vi "authorize summary.vi"(4 "error in (no error)":errorcluster, 6 "Authorization Request Sent? (f)":bool, 7 "Authorization":T2) -> (0 "error out":errorcluster, 3 "Template Keys":T1)   [LabVIEW 2011]
uses:
  license/Authorization Data.ctl
  ITK EXT/utils/keyedarr.llb/Keyed Array.ctl
  server/server lib/Spartan CONFIG Global.vi
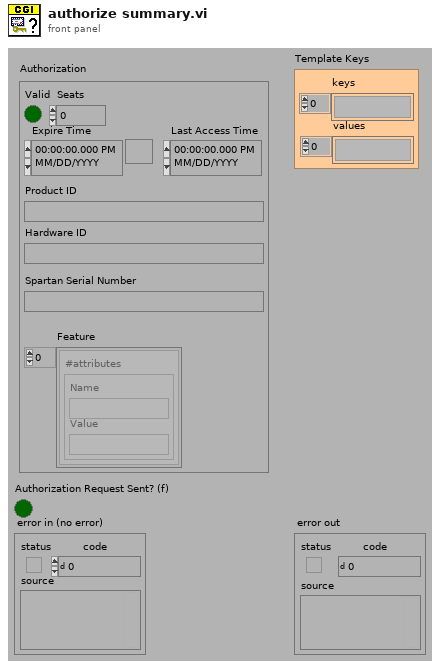
[diagram p1: front panel]
types:
  T1 = typedef "Keyed Array.ctl" = cluster{"keys":string[], "values":string[]}
  T2 = typedef "Authorization Data.ctl" = cluster{"Valid":bool, "Seats":i32, "Expire Time":timestamp, "Last Access Time":timestamp, "Product ID":string, "Hardware ID":string, "Spartan Serial Number":string, "Feature":cluster{"#attributes":cluster{"Name":string, "Value":string}}[]}
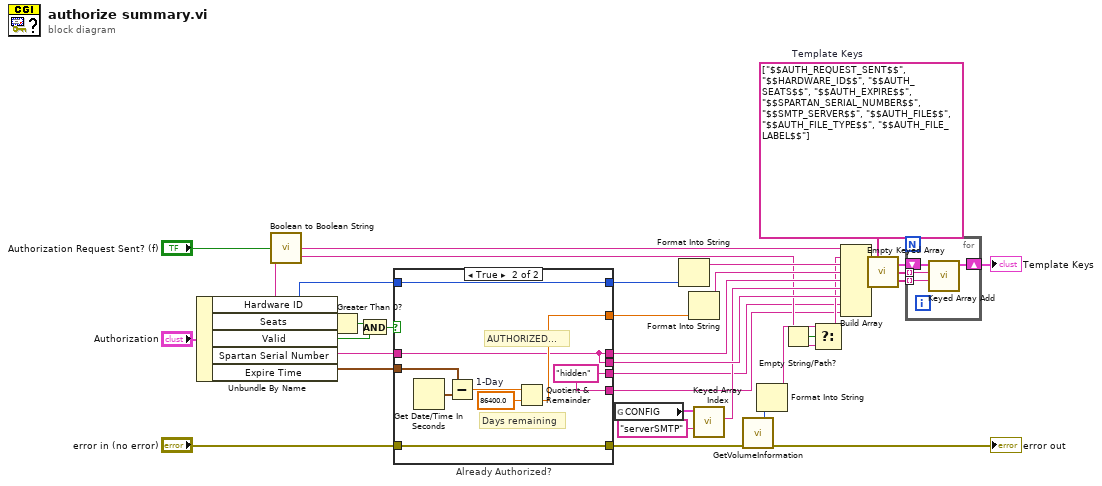
[diagram p0: block diagram]
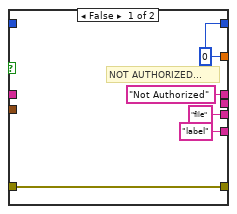
[diagram p2: hidden frame]
diagram:
  w30 = string[] ["$$AUTH_REQUEST_SENT$$", "$$HARDWARE_ID$$", "$$AUTH_SEATS$$", "$$AUTH_EXPIRE$$", "$$SPARTAN_SERIAL_NUMBER$$", "$$SMTP_SERVER$$", "$$AUTH_FILE$$", "$$AUTH_FILE_TYPE$$", "$$AUTH_FILE_LABEL$$"]  # Template Keys
  n1 = Unbundle By Name("Authorization") -> ("Hardware ID"=w4:string, "Seats"=w13:i32, "Valid"=w11:bool, "Spartan Serial Number"=w10:string, "Expire Time"=w14:timestamp)
  n2 = call "Boolean to Boolean String.vi"("Boolean"="Authorization Request Sent? (f)") -> ("Boolean string"=w26:string)  [unwired: 1 in]
  n3 = Greater Than 0?(x=w13) -> (x > 0?=w16:bool)
  n4 = And(x=w16, y=w11) -> (x .and. y?=w15:bool)
  n5 = case "Already Authorized?" shown="True" w15 {
    tunnel: "error in (no error)" -> [w37 w46]
    tunnel: [w37 w46] -> w7
    tunnel: [w35 w41] -> w24
    tunnel: ["Not Authorized" w39] -> w22
    tunnel: [_ w39] -> w20
    tunnel: w14 -> [_ w44]
    tunnel: w13 -> [_ w40]
    tunnel: [w35 w40] -> w12
    tunnel: w10 -> [_ w39]
    tunnel: ["file" ("key") w38] -> w2
    tunnel: ["label" ("key") w38] -> w1
    frame False {
      w35 = 0 ("Days/runs remaining")
      # "NOT AUTHORIZED..."
    }
    frame True {
      w38 = "hidden" ("key")
      w43 = 86400.0  # 1-Day
      # "Days remaining"
      # "AUTHORIZED..."
      n6 = Get Date/Time In Seconds() -> (seconds since 1Jan1904=w45:timestamp)
      n7 = Subtract(x=w44, y=w45) -> (x-y=w42:dbl)
      n8 = Quotient & Remainder(x=w42, y=w43) -> (floor(x/y)=w41:dbl)  [unwired: 1 out]
    }
  }
  n9 = global read "Spartan CONFIG Global.vi" "CONFIG"() -> (w19:T1)
  n10 = Format Into String(w12) -> (resulting string=w25:string)  [unwired: 3 in, 1 out]
  n11 = Format Into String(w24) -> (resulting string=w23:string)  [unwired: 3 in, 1 out]
  n12 = call "Keyed Array Index.vi"("key"="serverSMTP", "array in"=w19) -> ("value"=w17:string)  [unwired: 2 in, 3 out]
  n13 = call "GetVolumeInformation.vi"("error in (no error)"=w7) -> ("VolumeSerialNumber"=w9:u32, "error out"=→"error out":errorcluster)  [unwired: 8 in, 5 out]
  n14 = Format Into String(w9) -> (resulting string=w5:string)  [unwired: 3 in, 1 out]
  n15 = Empty String/Path?(string/path=w4) -> (empty?=w6:bool)
  n16 = Select(t=w5, s=w6, f=w4) -> (s? t:f=w3:string)
  n17 = Build Array(w26, w3, w25, w23, w22, w17, w20, w2, w1) -> (w29:string[])
  n18 = call "Empty Keyed Array.vi"() -> ("empty keyed array"=w28:T1)  [unwired: 3 out]
  n19 = for {
    tunnel: w30 -> [w50] mode=indexing
    tunnel: w29 -> [w49] mode=indexing
    shift-right: [w48] -> w27
    shift-left: w28 -> [w47]
    n20 = call "Keyed Array Add.vi"("value"=w49, "key"=w50, "array in"=w47) -> ("array out"=w48:T1)  [unwired: 1 in, 3 out]
  }
  "Template Keys" <- w27
